vi "M Hybrid car.vi"(11 "EV3 in":T1) -> (3 "EV3 out":T1)   [LabVIEW 2016]
uses:
  <vilib>/NXT/Subs/LVHSConnector.ctl
  <vilib>/NXT/LegoClasses/BrickReference/BrickReference.lvclass
  <vilib>/NXT/Dual Mode Library/Waits/Wait_Num(msec).vi
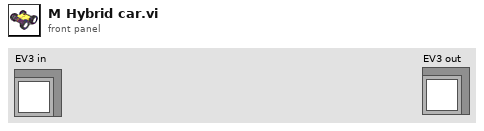
[diagram p1: front panel]
types:
  T1 = typedef "LVHSConnector.ctl" = refnum<class "BrickReference.lvclass">
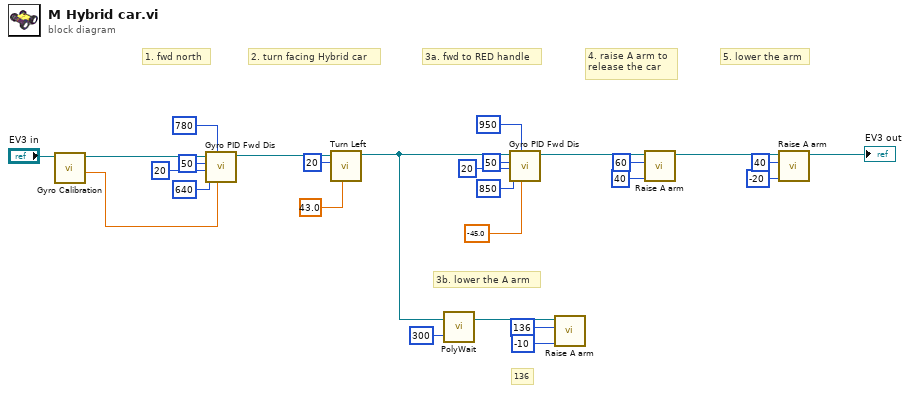
[diagram p0: block diagram]
diagram:
  # "136"
  # "5. lower the arm"
  # "4. raise A arm to \nrelease the car"
  # "3b. lower the A arm"
  # "3a. fwd to RED handle"
  # "2. turn facing Hybrid car"
  # "1. fwd north"
  n1 = call "Gyro Calibration.vi"("NXT/EV3"="EV3 in") -> ("Degrees"=w22:sgl, "NXT/EV3"=w27:T1)  [unwired: 6 in, 1 out]
  n2 = call "Gyro PID Fwd Dis.vi"("Target angle"=w22, "Threshold to stop"=780, "Threshold to slow"=640, "Min. speed"=20, "Max. speed"=50, "EV3 in"=w27) -> ("EV3 out"=w15:T1)  [unwired: 5 in]
  n3 = call "Turn Left.vi"("Turning angle"=sgl 43.0, "Motor B (right)"=i8 20, "EV3 in"=w15) -> ("EV3 out"=w11:T1)  [unwired: 8 in]
  n4 = call-poly <vilib>:"PolyWait.vi"("Time (100 msec)"=u32 300, "NXT/EV3"=w11) -> ("NXT/EV3"=w10:T1)  [unwired: 2 in]
  n5 = call "Gyro PID Fwd Dis.vi"("Target angle"=sgl -45.0, "Threshold to stop"=950, "Threshold to slow"=850, "Min. speed"=20, "Max. speed"=50, "EV3 in"=w11) -> ("EV3 out"=w6:T1)  [unwired: 5 in]
  n6 = call "Raise A arm.vi"("Power"=i8 -10, "Rotation"=136, "EV3 in"=w10) -> ()  [unwired: 8 in, 1 out]
  n7 = call "Raise A arm.vi"("Power"=i8 40, "Rotation"=60, "EV3 in"=w6) -> ("EV3 out"=w5:T1)  [unwired: 8 in]
  n8 = call "Raise A arm.vi"("Power"=i8 -20, "Rotation"=40, "EV3 in"=w5) -> ("EV3 out"=→"EV3 out":T1)  [unwired: 8 in]
